vi "Stop.vi"(8 "error in (no error)":errorcluster, 11 "Calibrator in":refnum<class "Calibrator.lvclass">) -> (0 "error out":errorcluster, 3 "Calibrator out":refnum<class "Calibrator.lvclass">)   [LabVIEW 2015, in "Calibrator.lvclass"]
uses:
  Calibrator.lvclass
  <instrlib>/Fluke 5XXX Series Multicalibrators/Fluke 5XXX Series Multicalibrators.lvlib
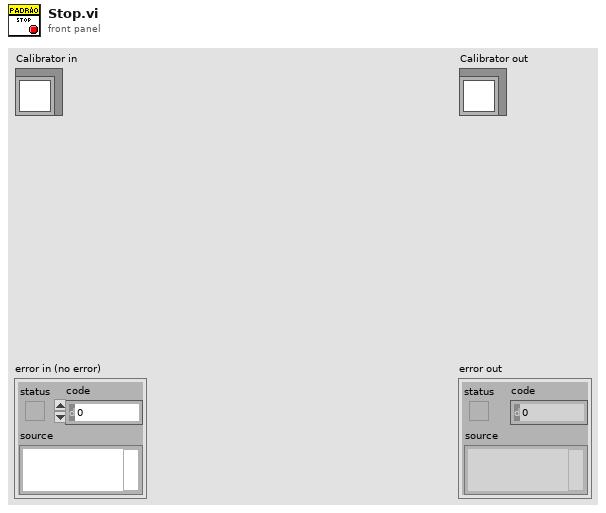
[diagram p1: front panel]
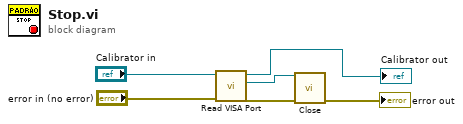
[diagram p0: block diagram]
diagram:
  n1 = call-dynamic "Read VISA Port.vi"("error in (no error)"="error in (no error)", "Device in"="Calibrator in") -> ("error out"=w1:errorcluster, "VISA Port"=w4:refnum<visa-resource-name>, "Device out"=→"Calibrator out":refnum<class "Calibrator.lvclass">)  [unwired: 7 in]
  n2 = call <instrlib>:"Close.vi"("VISA resource name"=w4, "error in (no error)"=w1) -> ("error out"=→"error out":errorcluster)  [unwired: 13 in]
